vi "power_transform.vi"(8 "error in":errorcluster caption="entrée d'erreur", 10 "X":string[][](array[string]), 11 "power_transform":T2={"method"="yeo-johnson", "standardize"=TRUE, "copy"=TRUE}) -> (0 "error out":errorcluster caption="sortie d'erreur", 3 "Data":T1)   [LabVIEW 2020]
doc: "Power transforms are a family of parametric, monotonic transformations that are applied to make data more Gaussian-like. This is useful for modeling issues related to heteroscedasticity (non-constant variance), or other situations where normality is desired.\n\nCurrently, power_transform supports the Box-Cox transform and the Yeo-Johnson transform. The optimal parameter for stabilizing variance and minimizing skewness is estimated through maximum likelihood.\n\nBox-Cox requires input data to be strictly positive, while Yeo-Johnson supports both positive or negative data.\n\nBy default, zero-mean, unit-variance normalization is applied to the transformed data.\n\n\nParameters :\n\n- X : array-like, shape (n_samples, n_features)\nThe data to be transformed using a power transformation.\n\n- method : {‘yeo-johnson’, ‘box-cox’}, default=’yeo-johnson’\nThe power transform method. Available methods are:\n\n‘yeo-johnson’, works with positive and negative values\n\n‘box-cox’, only works with strictly positive values\n\n- standardize : boolean, default=True\nSet to True to apply zero-mean, unit-variance normalization to the transformed output.\n\n- copy : boolean, optional, default=True\nSet to False to perform inplace computation during transformation.\n\nReturns : \n\n- X_trans : array-like, shape (n_samples, n_features)\nThe transformed data."
uses:
  power_transform.lvclass
panel:
  out "power_transform.lvclass":refnum<class "power_transform.lvclass">
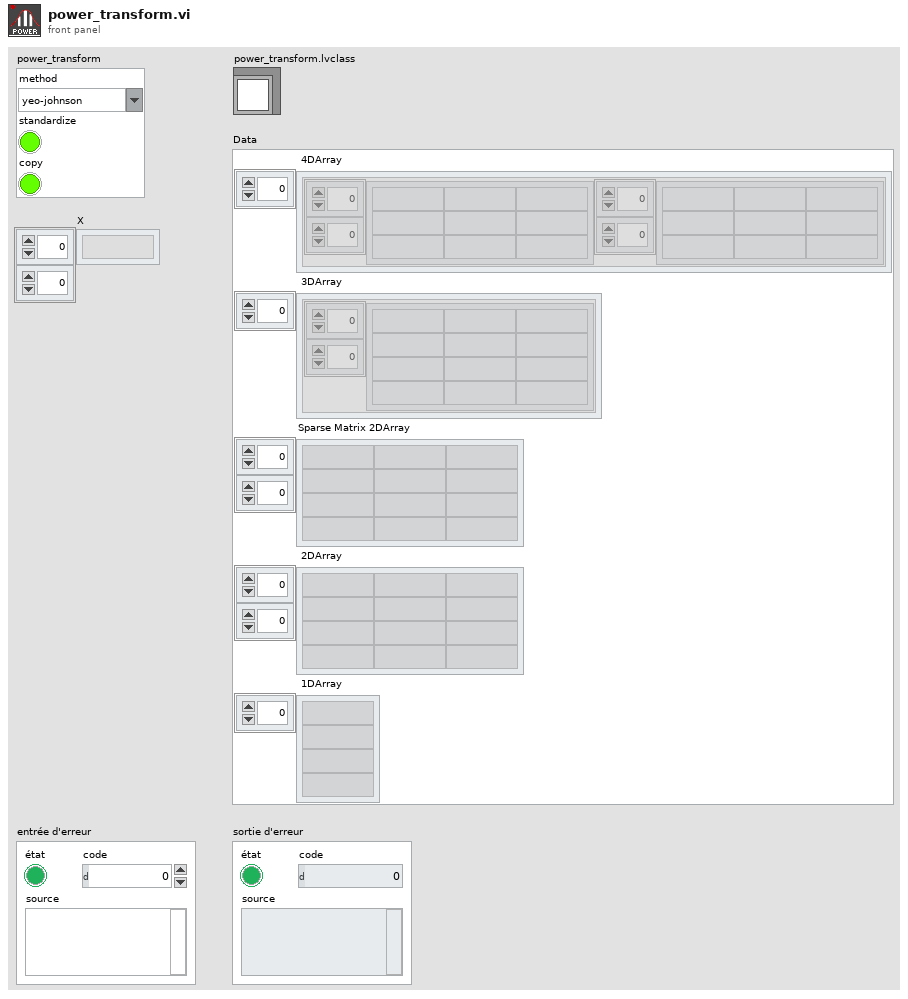
[diagram p1: front panel]
types:
  T1 = cluster{" 4DArray":cluster{"1":string[][], "2":string[][]}[], " 3DArray":cluster{"Tableau":string[][]}[], "Sparse Matrix 2DArray":string[][], " 2DArray":string[][], " 1DArray":string[]}
  T2 = cluster{"method":string, "standardize":bool, "copy":bool}
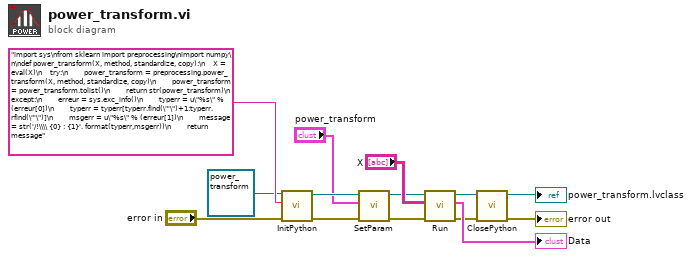
[diagram p0: block diagram]
diagram:
  n1 = call-dynamic "InitPython.vi"("error in (no error)"="error in", "Python Instruction"="import sys\nfrom sklearn import preprocessing\nimport numpy\n\ndef power_transform(X, method, standardize, copy):\n    X = eval(X)\n    try:\n        power_transform = preprocessing.power_transform(X, method, standardize, copy)\n        power_transform  = power_transform.tolist()\n        return str(power_transform)\n    except:\n        erreur = sys.exc_info()\n        typerr = u\"%s\" % (erreur[0])\n        typerr = typerr[typerr.find(\"'\")+1:typerr.rfind(\"'\")]\n        msgerr = u\"%s\" % (erreur[1])\n        message = str('/!\\\\ {0} : {1}'. format(typerr,msgerr))\n        return message", "Scikit-learn en entrée"=refnum<class "power_transform.lvclass"> refnum ("power_transform.lvclass")) -> ("error out"=w3:errorcluster, "Scikit-learn en sortie"=w5:refnum<class "power_transform.lvclass">)  [unwired: 7 in]
  n2 = call-dynamic "SetParam.vi"("error in (no error)"=w3, "power_transform"="power_transform", "power_transform.lvclass"=w5) -> ("error out"=w1:errorcluster, "power_transform.lvclass"=w2:refnum<class "power_transform.lvclass">)  [unwired: 7 in]
  n3 = call-dynamic "Run.vi"("error in (no error)"=w1, "X"="X", "power_transform.lvclass"=w2) -> ("error out"=w6:errorcluster, "Data"=→"Data":T1, "power_transform.lvclass"=w8:refnum<class "power_transform.lvclass">)  [unwired: 6 in]
  n4 = call-dynamic "ClosePython.vi"("error in (no error)"=w6, "Scikit-learn en entrée"=w8) -> ("error out"=→"error out":errorcluster, "Scikit-learn en sortie"=→"power_transform.lvclass":refnum<class "power_transform.lvclass">)  [unwired: 8 in]
